vi "Action Reset Alarms.vi"(0 "VISA resource name":refnum<visa-resource-name>, 7 "Reset Alarms (T: Reset Alarms)":bool=TRUE, 11 "error in (no error)":errorcluster) -> (4 "VISA resource name out":refnum<visa-resource-name>, 15 "error out":errorcluster)   [LabVIEW 2019, in "Lake Shore Cryotronics 340.lvlib"]
doc: "This VI clears both the high and low status of all alarms, including latching alarms."
uses:
  Lake Shore Cryotronics 340.lvlib
panel:
  # "Reset Alarms\nDo Not Reset Alarms"
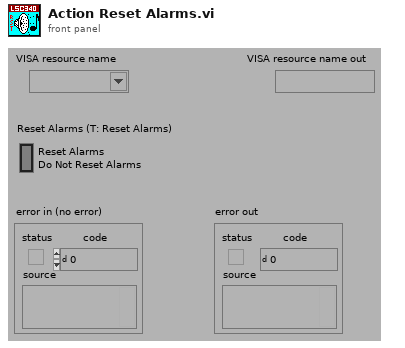
[diagram p1: front panel]
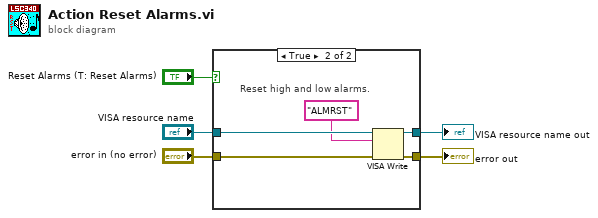
[diagram p0: block diagram]
diagram:
  n1 = case shown="True" "Reset Alarms (T: Reset Alarms)" {
    tunnel: "VISA resource name" -> [w7 w12]
    tunnel: "error in (no error)" -> [w6 w11]
    tunnel: [w7 w10] -> w1
    tunnel: [w6 w9] -> w2
    frame False {
      # "Do not reset alarms."
    }
    frame True {
      # "Reset high and low alarms."
      n2 = VISA Write(VISA resource name=w12, write buffer="ALMRST", error in (no error)=w11) -> (VISA resource name out=w10:refnum<visa-resource-name>, error out=w9:errorcluster)  [unwired: 1 out]
    }
  }
  "error out" <- w2
  "VISA resource name out" <- w1
